vi "Method 1.vi"(8 "error in (no error)":errorcluster, 10 "My Input":dbl, 11 "Test Actor 1 in":refnum<class "Test Actor 1.lvclass">) -> (0 "error out":errorcluster, 3 "Test Actor 1 out":refnum<class "Test Actor 1.lvclass">)   [LabVIEW 2023, in "Test Actor 1.lvlib" / "Test Actor 1.lvclass"]
doc: "My Method Description"
uses:
  Test Actor 1.lvclass
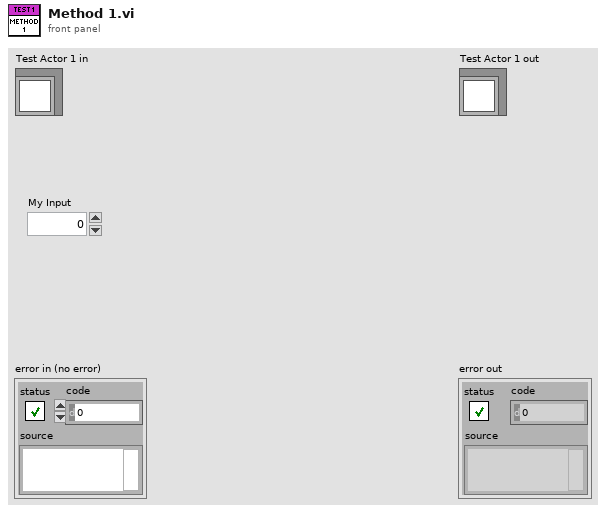
[diagram p1: front panel]
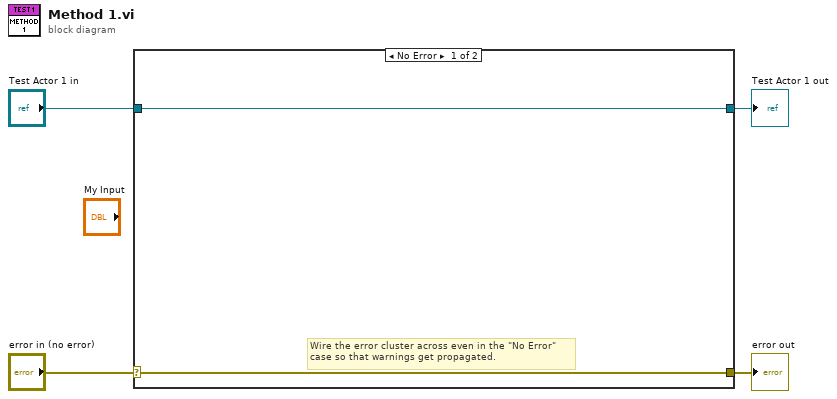
[diagram p0: block diagram]
diagram:
  n1 = case shown="No Error" "error in (no error)" {
    selector: "error in (no error)" -> [w5 w8]
    tunnel: [w5 w8] -> w3
    tunnel: [w6 w7] -> w1
    tunnel: "Test Actor 1 in" -> [w6 w7]
    frame No Error {
      # "Wire the error cluster across even in the \"No Error\"\ncase so that warnings get propagated."
    }
    frame Error {
    }
  }
  "error out" <- w3
  "Test Actor 1 out" <- w1
